vi "5. Cut Image from ROI.vi"() -> ()   [LabVIEW 2019]
doc: "c 2020 ReMiSYS All rights reserved."
uses:
  <vilib>/vision/NI_Vision_Development_Module.lvlib
panel:
  in  "Optional Rectangle":i32[](array[numeric])
  out "Global Rectangle":i32[](array[numeric])
  in  "Stop (F)":bool
  out "cut":T1(plugin-control)
  out "ori":T1(plugin-control)
  # "c 2022 ReMiSYS All rights reserved."
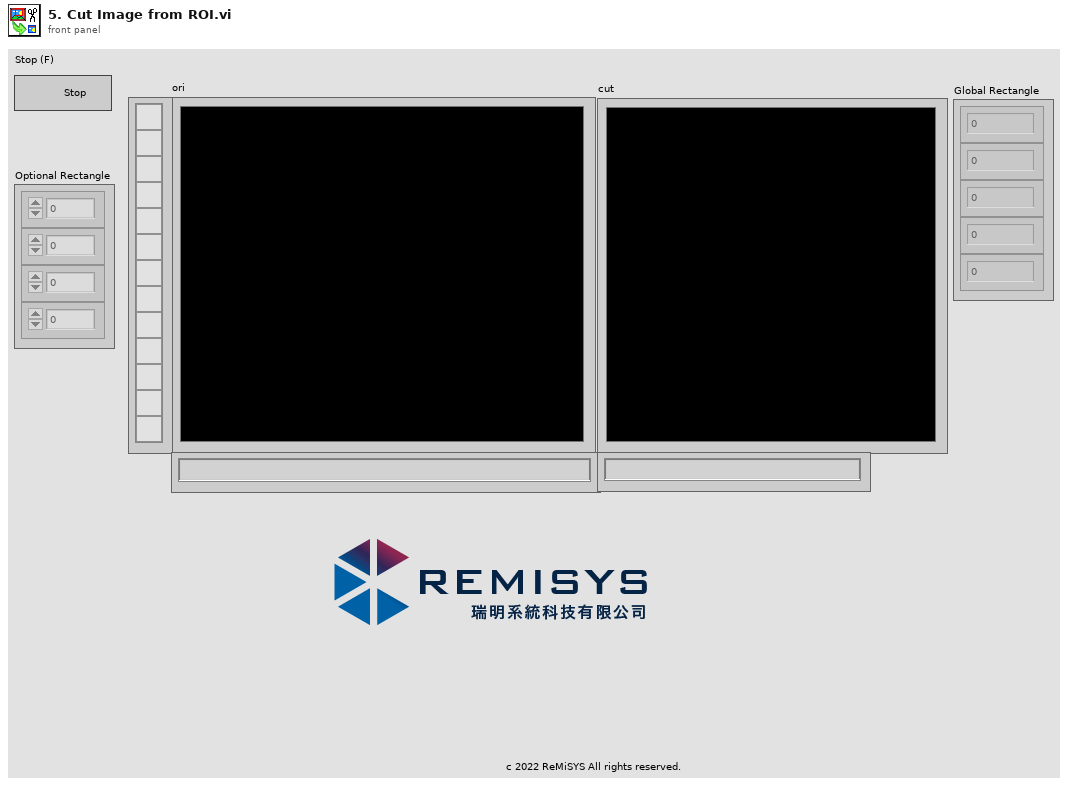
[diagram p1: front panel]
types:
  T1 = typedef "IMAQ Image.ctl" = refnum<image>
  T2 = typedef "Image Type" = u32
  T3 = cluster{"Global Rectangle":i32[], "Contours":cluster{"Contour Type":u32, "ROI Type":u32, "Points":i32[]}[]}
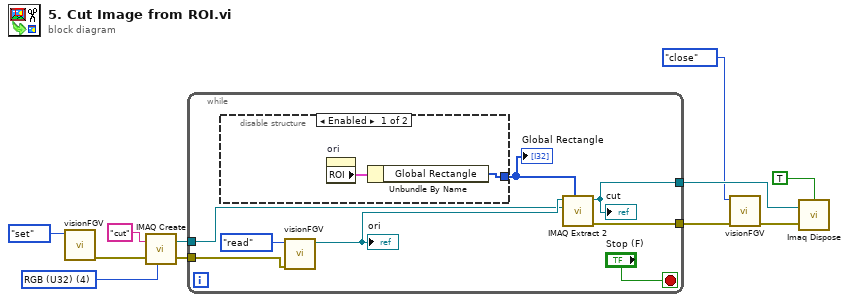
[diagram p0: block diagram]
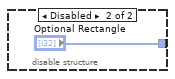
[diagram p2: hidden frame]
diagram:
  w8 = T2 4 items=["Grayscale (U8)", "Grayscale (I16)", "Grayscale (SGL)", "Complex (CSG)", "RGB (U32)", "HSL (U32)", "RGB (U64)", "Grayscale (U16)"] ("Image Type")
  n1 = call "visionFGV.vi"("Function"=enum16{"set", "read", "close"}."set") -> ("error out"=w4:errorcluster)  [unwired: 9 in, 1 out]
  n2 = call "IMAQ Create"("Image Name"="cut", "Image Type"=w8, "error in (no error)"=w4) -> ("New Image"=w9:T1, "error out"=w7:errorcluster)  [unwired: 2 in]
  n3 = while {
    tunnel: w9 -> [w17]
    tunnel: w7 -> [w19]
    tunnel: [w15] -> w6
    tunnel: [w12] -> w2
    stop <- "Stop (F)" stop-if-true
    n4 = disable-structure shown="Enabled" {
      disable-tunnel: [w20 "Optional Rectangle"] -> w16
      frame Enabled {
        n5 = property on="ori" class="ImageControl"() -> ("ROI"=w21:T3)  [unwired: 2 in, 2 out]
        n6 = Unbundle By Name(w21) -> ("Global Rectangle"=w20:i32[])
      }
      frame Disabled {
      }
    }
    "Global Rectangle" <- w16
    n7 = call "visionFGV.vi"("Error In"=w19, "Function"=enum16{"set", "read", "close"}."read") -> ("Image Out fgv"=w18:T1)  [unwired: 8 in, 1 out]
    "ori" <- w18
    n8 = call "IMAQ Extract 2"("Optional Rectangle"=w16, "Image Dst"=w17, "Image Src"=w18) -> ("error out"=w12:errorcluster, "Image Dst Out"=w15:T1)  [unwired: 7 in]
    "cut" <- w15
  }
  n9 = call "visionFGV.vi"("Error In"=w2, "Function"=enum16{"set", "read", "close"}."close") -> ("error out"=w3:errorcluster)  [unwired: 8 in, 1 out]
  n10 = call "Imaq Dispose"("All Images? (No)"=TRUE, "Image"=w6, "error in (no error)"=w3) -> ()  [unwired: 3 in, 1 out]
